vi "ImageSaveImage.vi"   [LabVIEW 2012, in "Image.lvclass"]
uses:
  classes/Image.lvclass
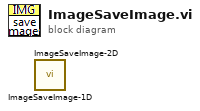
[diagram p0: block diagram]
diagram:
  n1 = call "ImageSaveImage-1D.vi"() -> ()  [unwired: 10 in, 2 out]
  n2 = call "ImageSaveImage-2D.vi"() -> ()  [unwired: 10 in, 2 out]
